vi "Move VI Image.vi"(7 "Images Destination":path=path "", 8 "Error In":errorcluster, 11 "VI Image File":path=path "") -> (0 "Error Out":errorcluster)   [LabVIEW 2018, in "Scripts.lvlib"]
uses:
  Scripts.lvlib
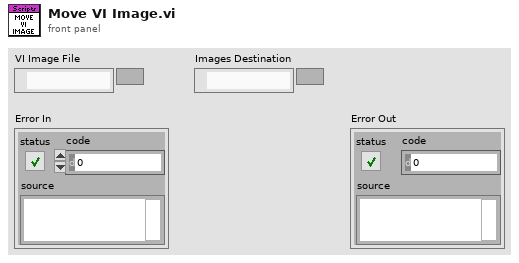
[diagram p1: front panel]
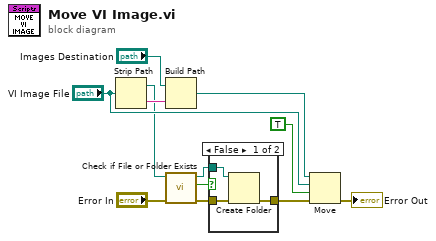
[diagram p0: block diagram]
diagram:
  n1 = Strip Path(path="VI Image File") -> (stripped path=w6:path, name=w7:string)
  n2 = Build Path(base path="Images Destination", name or relative path=w7) -> (appended path=w11:path)
  n3 = call <vilib>:"Check if File or Folder Exists.vi"("error in (no error)"="Error In", "path"=w6) -> ("error out"=w1:errorcluster, "file or folder exists?"=w4:bool, "dup path"=w5:path)  [unwired: 7 in]
  n4 = case shown="False" w4 {
    tunnel: w5 -> [w15 _]
    tunnel: [w14 w16] -> w3
    tunnel: w1 -> [w13 w16]
    frame False {
      n5 = Create Folder(path (use dialog)=w15, error in=w13) -> (error out=w14:errorcluster)  [unwired: 1 in, 2 out]
    }
    frame True {
    }
  }
  n6 = Move(source path=w11, error in=w3, 9:TRUE ("overwrite (F)"), 10:"VI Image File") -> (error out=→"Error Out":errorcluster)  [unwired: 1 in, 2 out]
